vi "ScaleRotAcc.vi"(6 "Scale Dir":T1=enum."Full scale -> Model scale", 8 "Scale factor":dbl, 11 "Rotational Acceleration (In)":dbl) -> (3 "Rotational Acceleration (Out)":dbl)   [LabVIEW 2018]
uses:
  Clusters/ScalingEnum.ctl
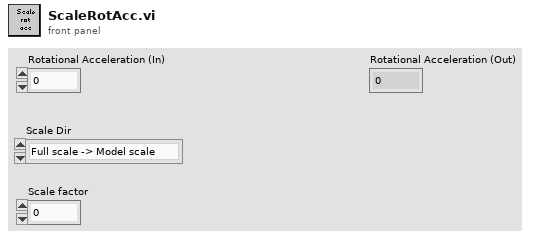
[diagram p1: front panel]
types:
  T1 = typedef "ScalingEnum.ctl" = enum16{"Model scale -> Full scale", "Full scale -> Model scale"}
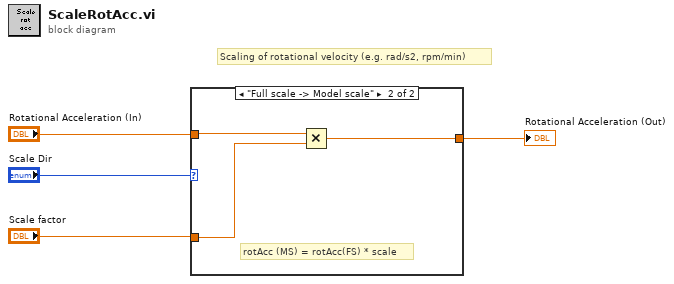
[diagram p0: block diagram]
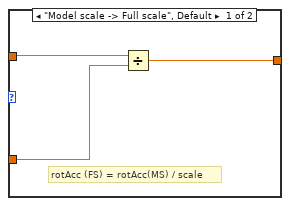
[diagram p2: hidden frame]
diagram:
  # "Scaling of rotational velocity (e.g. rad/s2, rpm/min)"
  n1 = case shown="\"Full scale -> Model scale\"" "Scale Dir" {
    tunnel: "Rotational Acceleration (In)" -> [w7 w10]
    tunnel: "Scale factor" -> [w6 w9]
    tunnel: [w5 w8] -> w1
    frame "Model scale -> Full scale", Default {
      # "rotAcc (FS) = rotAcc(MS) / scale"
      n2 = Divide(x=w7, y=w6) -> (x/y=w5:dbl)
    }
    frame "Full scale -> Model scale" {
      # "rotAcc (MS) = rotAcc(FS) * scale"
      n3 = Multiply(x=w10, y=w9) -> (x*y=w8:dbl)
    }
  }
  "Rotational Acceleration (Out)" <- w1
